vi "setRoi.vi"(0 "CCD in":refnum<class "CCD.lvclass">, 1 "ROI-index":i32=1, 3 "xSize":i32=1024, 4 "ySize":i32=256, 5 "error in (no error)":errorcluster, 7 "Delay between send and receive [ms]":i32=1000, 8 "xOrigin":i32, 9 "xBin":i32=1, 10 "yOrigin":i32, 11 "yBin":i32=256) -> (14 "CCD out":refnum<class "CCD.lvclass">, 15 "results-JSON string":string, 17 "ID":i32, 19 "error out":errorcluster)   [LabVIEW 2023, in "CCD.lvclass"]
uses:
  CCD.lvclass
  20f7d3bd-08ac-4524-9bed-df36c1da25a0.vi
  9c26a383-523e-4ef9-a52a-706f8f4d1e65.vi
  1afe4a3d-b8bf-4f9d-9cc3-ba347473a4dc.vi
  d2cc8e8b-a651-4a70-b231-21b727c34a88.vi
  78f3776e-fcd2-403b-b8de-9f13c4dda721.vi
  5b814308-78b1-4a9c-bf28-8cb0948429f0.vi
  78c51d80-a721-4af1-9d67-26e0a1c83448.vi
  dcdbc937-b8fd-44b7-ad82-9af9f3ab8d2e.vi
  <vilib>/JDP Science/JSONtext/Variant to JSON Text.vi
  <vilib>/JDP Science/JSONtext/Set Item.vi
  <vilib>/JDP Science/JSONtext/LVClass Serializer/JSONtext LVClass Serializer.lvclass
  GenericDevice/GenericDevice.lvclass
  <vilib>/IlluminatedG/lv-web-crypto/lv-json/JSON/JSON.lvlib
panel:
  # "Connector Pane"
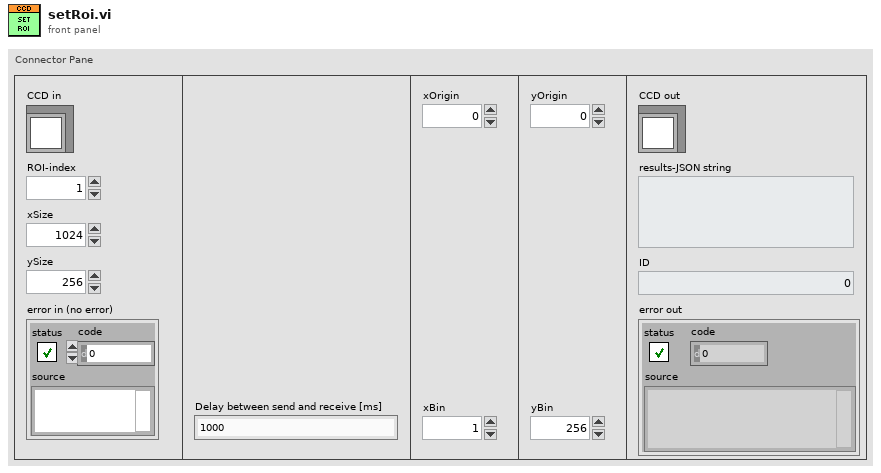
[diagram p1: front panel]
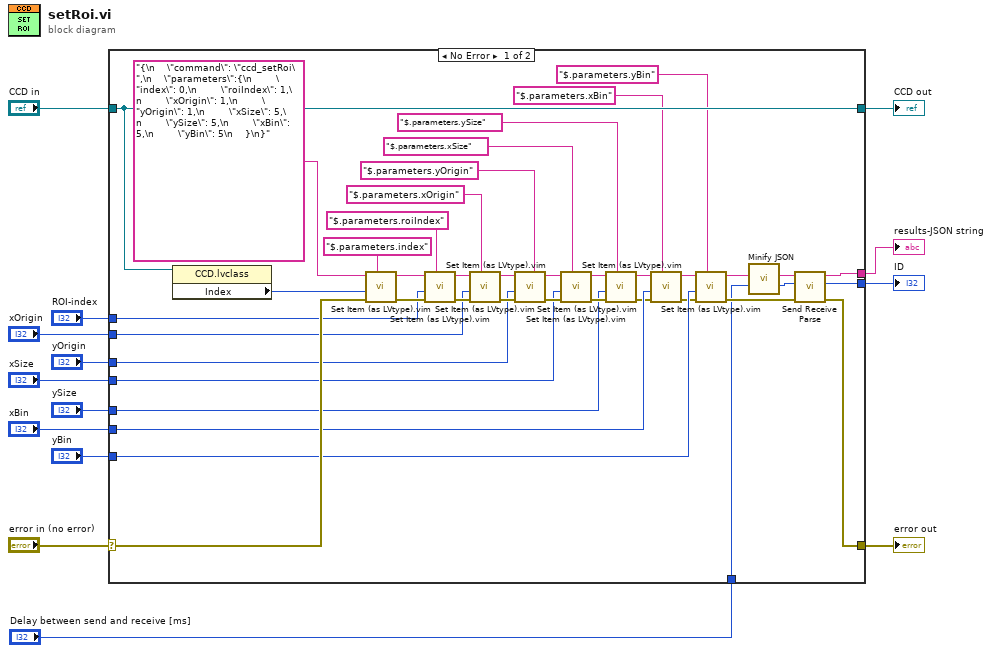
[diagram p0: block diagram]
diagram:
  n1 = case shown="No Error" "error in (no error)" {
    selector: "error in (no error)" -> [w50 w56]
    tunnel: [w18 w56] -> w13
    tunnel: [w52 w55] -> w11
    tunnel: "CCD in" -> [w52 w55]
    tunnel: "ROI-index" -> [w43 _]
    tunnel: "xOrigin" -> [w42 _]
    tunnel: "yOrigin" -> [w38 _]
    tunnel: "xSize" -> [w31 _]
    tunnel: "ySize" -> [w30 _]
    tunnel: "xBin" -> [w28 _]
    tunnel: "yBin" -> [w27 _]
    tunnel: [w20 _] -> w3
    tunnel: [w19 _] -> w2
    tunnel: "Delay between send and receive [ms]" -> [w15 _]
    frame No Error {
      n2 = property class="CCD.lvclass"(reference=w52) -> ("Index"=w51:i32)  [unwired: 1 in, 2 out]
      n3 = call "Set Item (as LVtype).vim"("$Path or Item Name"="$.parameters.index", "error in (no error)"=w50, "Anything"=w51, "JSON"="{\n    \"command\": \"ccd_setRoi\",\n    \"parameters\":{\n        \"index\": 0,\n        \"roiIndex\": 1,\n        \"xOrigin\": 1,\n        \"yOrigin\": 1,\n        \"xSize\": 5,\n        \"ySize\": 5,\n        \"xBin\": 5,\n        \"yBin\": 5\n    }\n}") -> ("error out"=w47:errorcluster, "<JSON>"=w48:string)  [unwired: 4 in, 1 out]
      n4 = call "Set Item (as LVtype).vim"("$Path or Item Name"="$.parameters.roiIndex", "error in (no error)"=w47, "Anything"=w43, "JSON"=w48) -> ("error out"=w45:errorcluster, "<JSON>"=w46:string)  [unwired: 4 in, 1 out]
      n5 = call "Set Item (as LVtype).vim"("$Path or Item Name"="$.parameters.xOrigin", "error in (no error)"=w45, "Anything"=w42, "JSON"=w46) -> ("error out"=w40:errorcluster, "<JSON>"=w39:string)  [unwired: 4 in, 1 out]
      n6 = call "Set Item (as LVtype).vim"("$Path or Item Name"="$.parameters.yOrigin", "error in (no error)"=w40, "Anything"=w38, "JSON"=w39) -> ("error out"=w34:errorcluster, "<JSON>"=w35:string)  [unwired: 4 in, 1 out]
      n7 = call "Set Item (as LVtype).vim"("$Path or Item Name"="$.parameters.xSize", "error in (no error)"=w34, "Anything"=w31, "JSON"=w35) -> ("error out"=w37:errorcluster, "<JSON>"=w36:string)  [unwired: 4 in, 1 out]
      n8 = call "Set Item (as LVtype).vim"("$Path or Item Name"="$.parameters.ySize", "error in (no error)"=w37, "Anything"=w30, "JSON"=w36) -> ("error out"=w25:errorcluster, "<JSON>"=w26:string)  [unwired: 4 in, 1 out]
      n9 = call "Set Item (as LVtype).vim"("$Path or Item Name"="$.parameters.xBin", "error in (no error)"=w25, "Anything"=w28, "JSON"=w26) -> ("error out"=w23:errorcluster, "<JSON>"=w29:string)  [unwired: 4 in, 1 out]
      n10 = call "Set Item (as LVtype).vim"("$Path or Item Name"="$.parameters.yBin", "error in (no error)"=w23, "Anything"=w27, "JSON"=w29) -> ("error out"=w24:errorcluster, "<JSON>"=w17:string)  [unwired: 4 in, 1 out]
      n11 = call <vilib>:"Minify JSON.vi"("JSON String"=w17) -> ("Minified JSON"=w16:string)  [unwired: 10 in]
      n12 = call "Send Receive Parse.vi"("error in"=w24, "Delay between send and receive [ms]"=w15, "<JSON>"=w16) -> ("error out"=w18:errorcluster, "ID"=w19:i32, "results-JSON string"=w20:string)  [unwired: 6 in]
    }
    frame Error {
    }
  }
  "error out" <- w13
  "CCD out" <- w11
  "results-JSON string" <- w3
  "ID" <- w2
